vi "GEOM_VAR_CustomKeys.vi"(6 "shdrsecs in":T1[](array[typedef])=[{"name"="TSEC", "directives"={"coords"="fpa", "reference"="phys", "xarea"="xdatastart:xdataend", "yarea"="ydatastart:ydataend", "order"="fits"}, "comment"="Good section from det _detID_  amp _ampID_", "amptype"=enum."ALL", "ampid"=TRUE, "detid"=TRUE, "unbin"=FALSE}, {"name"="ASEC", "directives"={"coords"="fpa", "reference"="pix", "xarea"="xdatastart:xdataend", "yarea"="ydatastart:ydataend", "order"="readout"}, "comment"="CCD  section in read order", "amptype"=enum."ALL", "ampid"=TRUE, "detid"=TRUE, "unbin"=FALSE}, {"name"="CSEC", "directives"={"coords"="fpa", "reference"="pix", "xarea"="xdatastart:xdataend", "yarea"="ydatastart:ydataend", "order"="fits"}, "comment"="CCD section from det _detID_  amp _ampID_", "amptype"=enum."ALL", "ampid"=TRUE, "detid"=TRUE, "unbin"=FALSE}, {"name"="BSEC", "directives"={"coords"="fpa", "reference"="phys", "xarea"="xposstart:xposend", "yarea"="ydatastart:ydataend", "order"="fits"}, "comment"="Overscan section from det _detID_  amp _ampID_", "amptype"=enum."ALL", "ampid"=TRUE, "detid"=TRUE, "unbin"=FALSE}, {"name"="DSEC", "directives"={"coords"="fpa", "reference"="phys", "xarea"="xdatastart:xdataend", "yarea"="ydatastart:ydataend", "order"="fits"}, "comment"="Data section from det _detID_  amp _ampID_", "amptype"=enum."ALL", "ampid"=TRUE, "detid"=TRUE, "unbin"=FALSE}], 8 "dethdrs in":T1[](array[typedef])=[{"name"="TRIMSEC", "directives"={"coords"="det", "reference"="phys", "xarea"="xdatastart:xdataend", "yarea"="ydatastart:ydataend", "order"="fits"}, "comment"="Good section from amp _ampID_", "amptype"=enum."ALL", "ampid"=TRUE, "detid"=FALSE, "unbin"=FALSE}, {"name"="DETSEC", "directives"={"coords"="fpa", "reference"="pix", "xarea"="xdatastart:xdataend", "yarea"="ydatastart:ydataend", "order"="fits"}, "comment"="Detector display tile", "amptype"=enum."ALL", "ampid"=TRUE, "detid"=FALSE, "unbin"=FALSE}, {"name"="CCDSEC", "directives"={"coords"="det", "reference"="pix", "xarea"="xdatastart:xdataend", "yarea"="ydatastart:ydataend", "order"="fits"}, "comment"="CCD section from _ampID_", "amptype"=enum."ALL", "ampid"=TRUE, "detid"=FALSE, "unbin"=FALSE}, {"name"="AMPSEC", "directives"={"coords"="det", "reference"="pix", "xarea"="xdatastart:xdataend", "yarea"="ydatastart:ydataend", "order"="readout"}, "comment"="CCD section in read order", "amptype"=enum."ALL", "ampid"=TRUE, "detid"=FALSE, "unbin"=FALSE}, {"name"="DATASEC", "directives"={"coords"="det", "reference"="phys", "xarea"="xdatastart:xdataend", "yarea"="ydatastart:ydataend", "order"="fits"}, "comment"="Data section from amp _ampID_", "amptype"=enum."ALL", "ampid"=TRUE, "detid"=FALSE, "unbin"=FALSE}, {"name"="BIASSEC", "directives"={"coords"="fpa", "reference"="phys", "xarea"="xposstart:xposend", "yarea"="ydatastart:ydataend", "order"="fits"}, "comment"="Overscan from _ampID_", "amptype"=enum."ALL", "ampid"=TRUE, "detid"=FALSE, "unbin"=FALSE}, {"name"="PRESEC", "directives"={"coords"="det", "reference"="phys", "xarea"="xprestart:xpreend", "yarea"="ydatastart:ydataend", "order"="fits"}, "comment"="Prescan from amp _ampID_", "amptype"=enum."ALL", "ampid"=TRUE, "detid"=FALSE, "unbin"=FALSE}, {"name"="POSTSEC", "directives"={"coords"="det", "reference"="phys", "xarea"="xdatastart:xdataend", "yarea"="yposstart:yposend", "order"="fits"}, "comment"="Postscan from amp _ampID_", "amptype"=enum."ALL", "ampid"=TRUE, "detid"=FALSE, "unbin"=FALSE}], 9 "Action":T4, 10 "format":T3={"inienclose"="[", "endenclose"="]", "rangesep"=":", "secsep"=","}, 11 "amphdrs in":T1[](array[typedef])=[{"name"="TRIMSEC", "directives"={"coords"="amp", "reference"="phys", "xarea"="xdatastart:xdataend", "yarea"="ydatastart:ydataend", "order"="fits"}, "comment"="Good section", "amptype"=enum."ALL", "ampid"=FALSE, "detid"=FALSE, "unbin"=FALSE}, {"name"="DETSEC", "directives"={"coords"="fpa", "reference"="pix", "xarea"="xdatastart:xdataend", "yarea"="ydatastart:ydataend", "order"="fits"}, "comment"="Detector display tile", "amptype"=enum."ALL", "ampid"=FALSE, "detid"=FALSE, "unbin"=FALSE}, {"name"="CCDSEC", "directives"={"coords"="det", "reference"="pix", "xarea"="xdatastart:xdataend", "yarea"="ydatastart:ydataend", "order"="fits"}, "comment"="CCD section to display", "amptype"=enum."ALL", "ampid"=FALSE, "detid"=FALSE, "unbin"=FALSE}, {"name"="AMPSEC", "directives"={"coords"="amp", "reference"="pix", "xarea"="xdatastart:xdataend", "yarea"="ydatastart:ydataend", "order"="readout"}, "comment"="CCD section in read order", "amptype"=enum."ALL", "ampid"=FALSE, "detid"=FALSE, "unbin"=FALSE}, {"name"="DATASEC", "directives"={"coords"="amp", "reference"="phys", "xarea"="xdatastart:xdataend", "yarea"="ydatastart:ydataend", "order"="fits"}, "comment"="Data section to display", "amptype"=enum."ALL", "ampid"=FALSE, "detid"=FALSE, "unbin"=FALSE}, {"name"="BIASSEC", "directives"={"coords"="amp", "reference"="phys", "xarea"="xposstart:xposend", "yarea"="ydatastart:ydataend", "order"="fits"}, "comment"="Overscan", "amptype"=enum."ALL", "ampid"=FALSE, "detid"=FALSE, "unbin"=FALSE}, {"name"="PRESEC", "directives"={"coords"="amp", "reference"="phys", "xarea"="xprestart:xpreend", "yarea"="ydatastart:ydataend", "order"="fits"}, "comment"="Prescan", "amptype"=enum."ALL", "ampid"=FALSE, "detid"=FALSE, "unbin"=FALSE}, {"name"="POSTSEC", "directives"={"coords"="amp", "reference"="phys", "xarea"="xdatastart:xdataend", "yarea"="yposstart:yposend", "order"="fits"}, "comment"="Postscan", "amptype"=enum."ALL", "ampid"=FALSE, "detid"=FALSE, "unbin"=FALSE}]) -> (0 "dethdrs out":T1[](array[typedef])=[{"name"="TRIMSEC", "directives"={"coords"="det", "reference"="phys", "xarea"="xdatastart:xdataend", "yarea"="ydatastart:ydataend", "order"="fits"}, "comment"="Good section from amp _ampID_", "amptype"=enum."ALL", "ampid"=TRUE, "detid"=FALSE, "unbin"=FALSE}, {"name"="DETSEC", "directives"={"coords"="fpa", "reference"="pix", "xarea"="xdatastart:xdataend", "yarea"="ydatastart:ydataend", "order"="fits"}, "comment"="Detector display tile", "amptype"=enum."ALL", "ampid"=TRUE, "detid"=FALSE, "unbin"=FALSE}, {"name"="CCDSEC", "directives"={"coords"="det", "reference"="pix", "xarea"="xdatastart:xdataend", "yarea"="ydatastart:ydataend", "order"="fits"}, "comment"="CCD section from _ampID_", "amptype"=enum."ALL", "ampid"=TRUE, "detid"=FALSE, "unbin"=FALSE}, {"name"="AMPSEC", "directives"={"coords"="det", "reference"="pix", "xarea"="xdatastart:xdataend", "yarea"="ydatastart:ydataend", "order"="readout"}, "comment"="CCD section in read order", "amptype"=enum."ALL", "ampid"=TRUE, "detid"=FALSE, "unbin"=FALSE}, {"name"="DATASEC", "directives"={"coords"="det", "reference"="phys", "xarea"="xdatastart:xdataend", "yarea"="ydatastart:ydataend", "order"="fits"}, "comment"="Data section from amp _ampID_", "amptype"=enum."ALL", "ampid"=TRUE, "detid"=FALSE, "unbin"=FALSE}, {"name"="BIASSEC", "directives"={"coords"="fpa", "reference"="phys", "xarea"="xposstart:xposend", "yarea"="ydatastart:ydataend", "order"="fits"}, "comment"="Overscan from _ampID_", "amptype"=enum."ALL", "ampid"=TRUE, "detid"=FALSE, "unbin"=FALSE}, {"name"="PRESEC", "directives"={"coords"="det", "reference"="phys", "xarea"="xprestart:xpreend", "yarea"="ydatastart:ydataend", "order"="fits"}, "comment"="Prescan from amp _ampID_", "amptype"=enum."ALL", "ampid"=TRUE, "detid"=FALSE, "unbin"=FALSE}, {"name"="POSTSEC", "directives"={"coords"="det", "reference"="phys", "xarea"="xdatastart:xdataend", "yarea"="yposstart:yposend", "order"="fits"}, "comment"="Postscan from amp _ampID_", "amptype"=enum."ALL", "ampid"=TRUE, "detid"=FALSE, "unbin"=FALSE}], 1 "shdrs out":T1[](array[typedef]), 2 "format out":T3={"inienclose"="[", "endenclose"="]", "rangesep"=":", "secsep"=","}, 3 "amphdrs out":T1[](array[typedef])=[{"name"="TRIMSEC", "directives"={"coords"="amp", "reference"="phys", "xarea"="xdatastart:xdataend", "yarea"="ydatastart:ydataend", "order"="fits"}, "comment"="Good section", "amptype"=enum."ALL", "ampid"=FALSE, "detid"=FALSE, "unbin"=FALSE}, {"name"="DETSEC", "directives"={"coords"="fpa", "reference"="pix", "xarea"="xdatastart:xdataend", "yarea"="ydatastart:ydataend", "order"="fits"}, "comment"="Detector display tile", "amptype"=enum."ALL", "ampid"=FALSE, "detid"=FALSE, "unbin"=FALSE}, {"name"="CCDSEC", "directives"={"coords"="det", "reference"="pix", "xarea"="xdatastart:xdataend", "yarea"="ydatastart:ydataend", "order"="fits"}, "comment"="CCD section to display", "amptype"=enum."ALL", "ampid"=FALSE, "detid"=FALSE, "unbin"=FALSE}, {"name"="AMPSEC", "directives"={"coords"="amp", "reference"="pix", "xarea"="xdatastart:xdataend", "yarea"="ydatastart:ydataend", "order"="readout"}, "comment"="CCD section in read order", "amptype"=enum."ALL", "ampid"=FALSE, "detid"=FALSE, "unbin"=FALSE}, {"name"="DATASEC", "directives"={"coords"="amp", "reference"="phys", "xarea"="xdatastart:xdataend", "yarea"="ydatastart:ydataend", "order"="fits"}, "comment"="Data section to display", "amptype"=enum."ALL", "ampid"=FALSE, "detid"=FALSE, "unbin"=FALSE}, {"name"="BIASSEC", "directives"={"coords"="amp", "reference"="phys", "xarea"="xposstart:xposend", "yarea"="ydatastart:ydataend", "order"="fits"}, "comment"="Overscan", "amptype"=enum."ALL", "ampid"=FALSE, "detid"=FALSE, "unbin"=FALSE}, {"name"="PRESEC", "directives"={"coords"="amp", "reference"="phys", "xarea"="xprestart:xpreend", "yarea"="ydatastart:ydataend", "order"="fits"}, "comment"="Prescan", "amptype"=enum."ALL", "ampid"=FALSE, "detid"=FALSE, "unbin"=FALSE}, {"name"="POSTSEC", "directives"={"coords"="amp", "reference"="phys", "xarea"="xdatastart:xdataend", "yarea"="yposstart:yposend", "order"="fits"}, "comment"="Postscan", "amptype"=enum."ALL", "ampid"=FALSE, "detid"=FALSE, "unbin"=FALSE}])   [LabVIEW 2016]
uses:
  GEOM_VAR_action.ctl
  Headers/GEOM_FormatGeomkeys.ctl
  Headers/GEOM_HdrSec.ctl
  Headers/GEOM_CoorSys.ctl
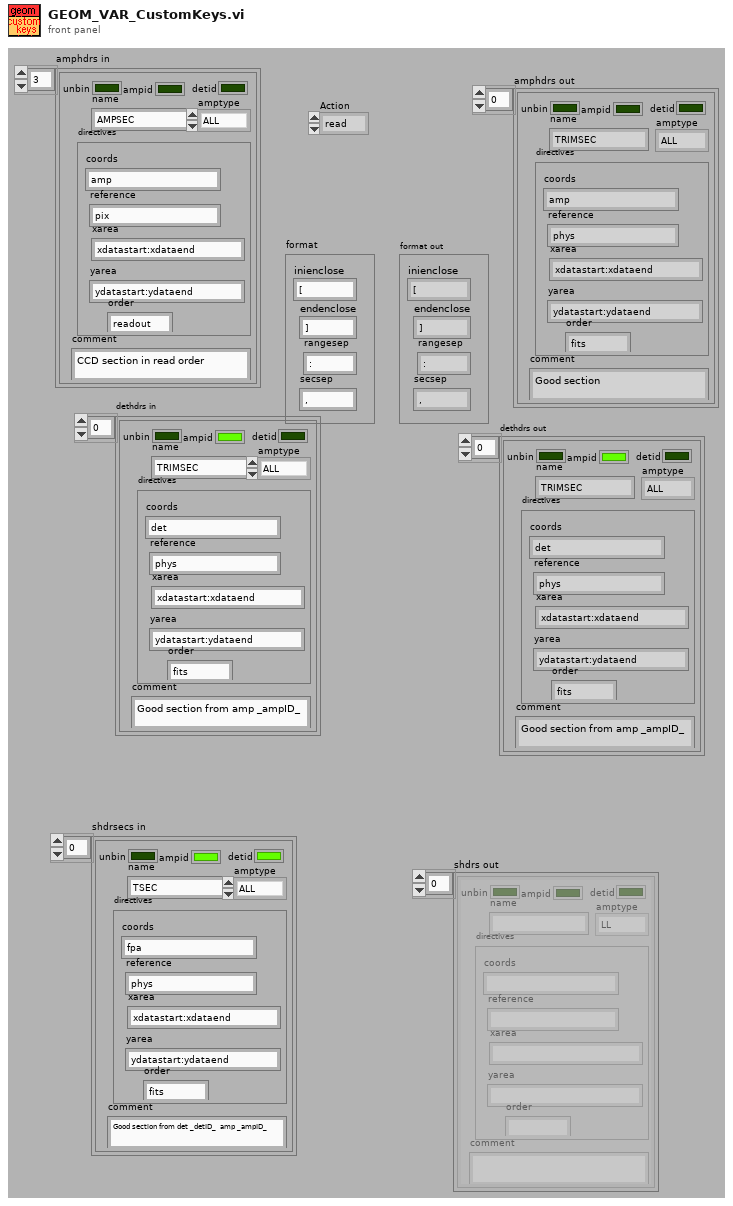
[diagram p1: front panel]
types:
  T1 = typedef "GEOM_HdrSec.ctl" = cluster{"name":string, "directives":T2, "comment":string, "amptype":enum16{"LL", "LR", "UL", "UR", "ALL", "LEFT", "RIGHT", "UPPER", "LOWER"}, "ampid":bool, "detid":bool, "unbin":bool}
  T2 = typedef "GEOM_CoorSys.ctl" = cluster{"coords":string, "reference":string, "xarea":string, "yarea":string, "order":string}
  T3 = typedef "GEOM_FormatGeomkeys.ctl" = cluster{"inienclose":string, "endenclose":string, "rangesep":string, "secsep":string}
  T4 = typedef "GEOM_VAR_action.ctl" = enum16{"read", "write"}
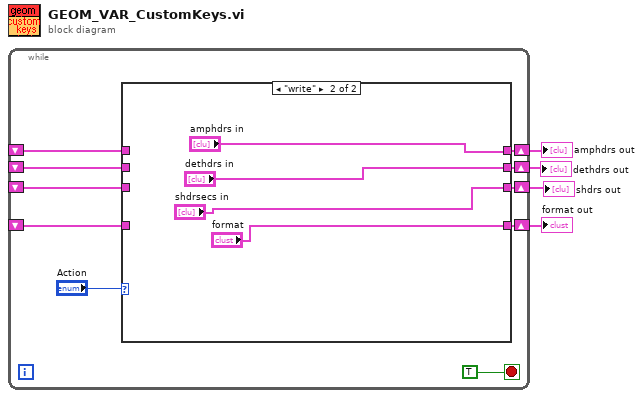
[diagram p0: block diagram]
diagram:
  n1 = while {
    shift-right: [w13] -> w3
    shift-left: _ -> [w12]
    shift-right: [w10] -> w4
    shift-left: _ -> [w9]
    shift-right: [w8] -> w2
    shift-left: _ -> [w6]
    shift-right: [w7] -> w1
    shift-left: _ -> [w5]
    stop <- TRUE stop-if-true
    n2 = case shown="\"write\"" "Action" {
      tunnel: [w18 "amphdrs in"] -> w13
      tunnel: w12 -> [w18 _]
      tunnel: [w17 "format"] -> w10
      tunnel: w9 -> [w17 _]
      tunnel: [w16 "dethdrs in"] -> w8
      tunnel: [w15 "shdrsecs in"] -> w7
      tunnel: w6 -> [w16 _]
      tunnel: w5 -> [w15 _]
      frame "read", Default {
      }
      frame "write" {
      }
    }
  }
  "format out" <- w4
  "amphdrs out" <- w3
  "dethdrs out" <- w2
  "shdrs out" <- w1
